vi "SwapValve.vi"(8 "Valve 2":i32, 11 "Valve 1":i32) -> ()   [LabVIEW 2011]
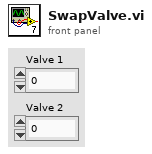
[diagram p1: front panel]
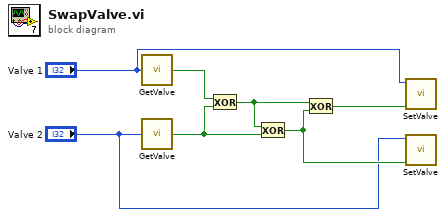
[diagram p0: block diagram]
diagram:
  n1 = call "GetValve.vi"("Numeric"="Valve 1") -> ("Boolean"=w7:bool)
  n2 = call "GetValve.vi"("Numeric"="Valve 2") -> ("Boolean"=w6:bool)
  n3 = Exclusive Or(1:w6, 2:w7) -> (0:w5:bool)
  n4 = Exclusive Or(1:w6, 2:w5) -> (0:w2:bool)
  n5 = Exclusive Or(1:w2, 2:w5) -> (0:w4:bool)
  n6 = call "SetValve.vi"("Open/Close"=w4, "Valve"="Valve 1") -> ()  [unwired: 10 in]
  n7 = call "SetValve.vi"("Open/Close"=w2, "Valve"="Valve 2") -> ()  [unwired: 10 in]
